vi "CreateNIPhysicalNameArrays.vi"() -> (0 "DAQ Array":string[][](array[string]), 1 "Timing Array":string[][](array[string]))   [LabVIEW 2013]
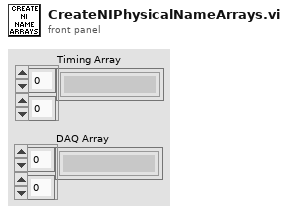
[diagram p1: front panel]
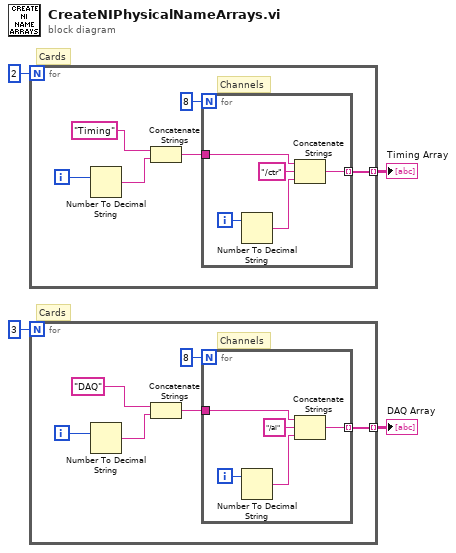
[diagram p0: block diagram]
diagram:
  # "Cards"
  # "Cards"
  n1 = for {
    N: 2 -> [_]
    tunnel: [w5] -> w3 mode=indexing
    i -> [w10]
    # "Channels"
    n2 = Number To Decimal String(number=w10) -> (decimal integer string=w9:string)  [unwired: 1 in]
    n3 = Concatenate Strings("Timing", w9) -> (w7:string)
    n4 = for {
      N: 8 -> [_]
      tunnel: w7 -> [w14]
      tunnel: [w11] -> w5 mode=indexing
      i -> [w13]
      n5 = Number To Decimal String(number=w13) -> (decimal integer string=w12:string)  [unwired: 1 in]
      n6 = Concatenate Strings(w14, "/ctr" ("string"), w12) -> (w11:string)
    }
  }
  "Timing Array" <- w3
  n7 = for {
    N: 3 -> [_]
    tunnel: [w16] -> w1 mode=indexing
    i -> [w21]
    # "Channels"
    n8 = Number To Decimal String(number=w21) -> (decimal integer string=w20:string)  [unwired: 1 in]
    n9 = Concatenate Strings("DAQ", w20) -> (w18:string)
    n10 = for {
      N: 8 -> [_]
      tunnel: w18 -> [w25]
      tunnel: [w22] -> w16 mode=indexing
      i -> [w24]
      n11 = Number To Decimal String(number=w24) -> (decimal integer string=w23:string)  [unwired: 1 in]
      n12 = Concatenate Strings(w25, "/ai" ("string"), w23) -> (w22:string)
    }
  }
  "DAQ Array" <- w1
